vi "HART_read_modbus_register.vi"(0 "port number":refnum<visa-resource-name>, 1 "Max listen time\n(1000 ms)":u32=1000, 5 "address (array)":u8[](array[numeric]), 9 "MODBUS Reg.":u16=162, 11 "error IN":errorcluster, 12 "data type":T2(ring), 13 "Byte order":T1(ring)=enum."2-3-0-1") -> (2 "Data bytes":u8[](array[numeric]) format="%.0x", 3 "raw response":u8[](array[numeric]) format="%.0x", 4 "Unsigned 16 out":u16, 6 "unsigned 32 out":u32, 8 "raw write":u8[](array[numeric]) format="%.0x", 10 "floating point out":sgl format="%#.6f", 14 "coil value":u8, 15 "error out":errorcluster)   [LabVIEW 2016]
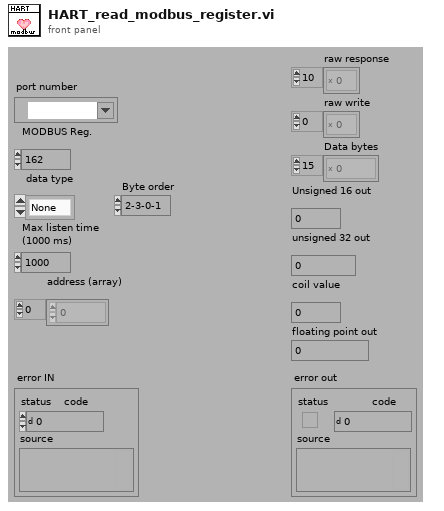
[diagram p1: front panel]
types:
  T1 = enum16{"0-1-2-3", "2-3-0-1", "1-0-3-2", "3-2-1-0"}
  T2 = enum16{"None", "Coil", "Uint16", "Uint32", "Float", "Undefined"}
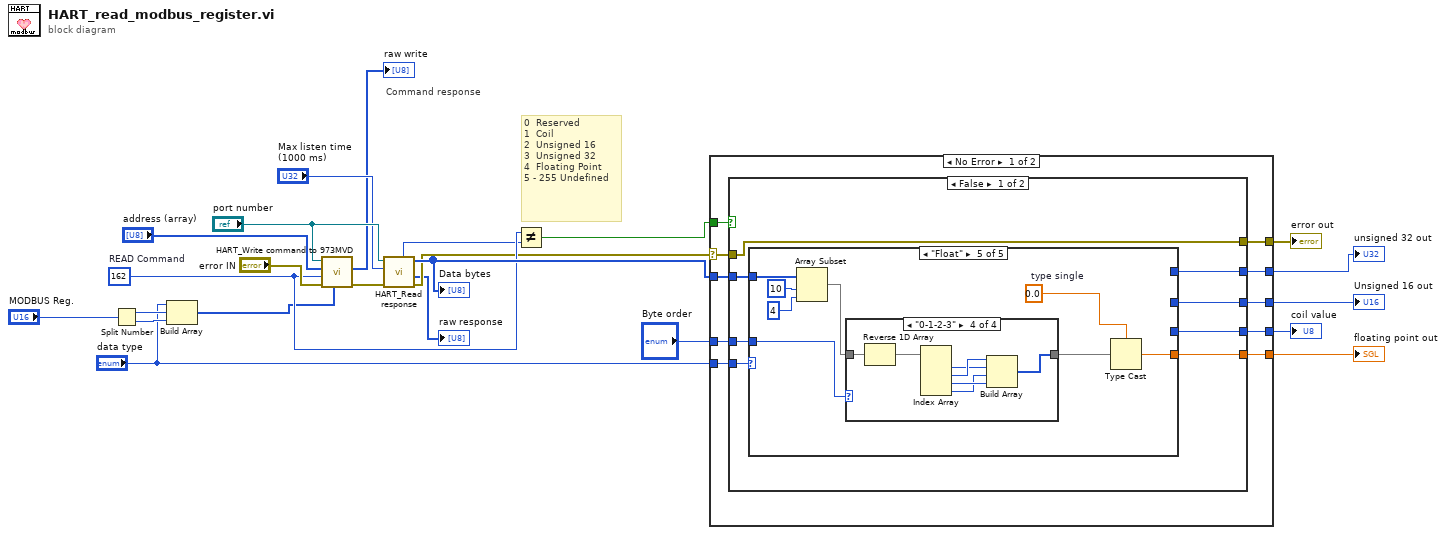
[diagram p0: block diagram]
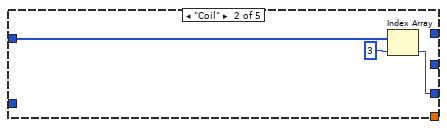
[diagram p3: hidden frame]
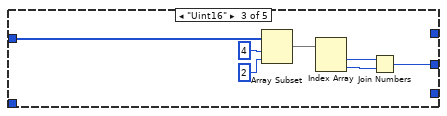
[diagram p4: hidden frame]
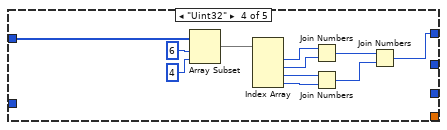
[diagram p5: hidden frame]
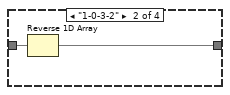
[diagram p7: hidden frame]
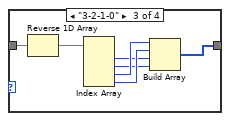
[diagram p8: hidden frame]
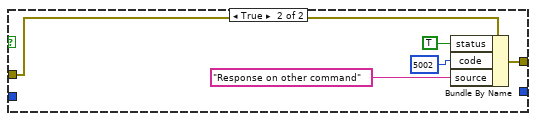
[diagram p9: hidden frame]
diagram:
  w19 = u8 162  # READ Command
  # "0\t\tReserved\n1\t\tCoil\n2\t\tUnsigned 16\n3\t\tUnsigned 32\n4\t\tFloating Point\n5 - 255\tUndefined"
  # "Command response"
  n1 = Split Number(x="MODBUS Reg.") -> (hi(x)=w13:u8, lo(x)=w12:u8)
  n2 = Build Array("data type", w13, w12) -> (w11:u16[])
  n3 = call "HART_Write command to 973MVD.vi"("data"=w11, "error in"="error IN", "READ Command"=w19, "address (array)"="address (array)", "resource name"="port number") -> ("error out"=w23:errorcluster, "appended array"=→"raw write":u8[])  [unwired: 5 in]
  n4 = call "HART_Read response.vi"("error in"=w23, "Max listen time\n(1000 ms)"="Max listen time\n(1000 ms)", "resource name"="port number") -> ("error out"=w16:errorcluster, "unsigned byte array"=→"raw response":u8[], "Data bytes"=w21:u8[], "Respons on\nCommand"=w18:u8)  [unwired: 3 in, 2 out]
  "Data bytes" <- w21
  n5 = Not Equal?(x=w19, y=w18) -> (x != y?=w20:bool)
  n6 = case shown="No Error" w16 {
    selector: w16 -> [w31 w93]
    tunnel: w21 -> [w33 _]
    tunnel: w20 -> [w32 _]
    tunnel: "data type" -> [w30 _]
    tunnel: [w29 w93] -> w10
    tunnel: [w28 _] -> w9
    tunnel: [w27 _] -> w8
    tunnel: [w26 _] -> w7
    tunnel: [w25 _] -> w6
    tunnel: "Byte order" -> [w24 _]
    frame No Error {
      n7 = case shown="False" w32 {
        tunnel: w33 -> [w40 _]
        tunnel: w31 -> [w39 w89]
        tunnel: [w39 w88] -> w29
        tunnel: w30 -> [w41 _]
        tunnel: [w38 _] -> w28
        tunnel: [w37 _] -> w27
        tunnel: [w36 _] -> w26
        tunnel: [w35 _] -> w25
        tunnel: w24 -> [w34 _]
        frame False {
          n8 = case shown="\"Float\"" w41 {
            tunnel: w40 -> [_ w44 w51 w62 w70]
            tunnel: [_ _ w45 _ _] -> w38
            tunnel: [_ _ _ w52 _] -> w37
            tunnel: [_ w42 _ _ _] -> w36
            tunnel: [_ _ _ _ w67] -> w35
            tunnel: w34 -> [_ _ _ _ w64]
            frame "None", Default {
            }
            frame "Coil" {
              n9 = Index Array(array=w44, index=3) -> (element=w42:u8)
            }
            frame "Uint16" {
              n10 = Array Subset(array=w51, index=4, length=2) -> (w48:u8[])
              n11 = Index Array(array=w48) -> (element #1=w47:u8, element #2=w46:u8)  [unwired: 2 in]
              n12 = Join Numbers(hi=w47, lo=w46) -> ((hi.lo)=w45:u16)
            }
            frame "Uint32" {
              n13 = Array Subset(array=w62, index=6, length=4) -> (w59:u8[])
              n14 = Index Array(array=w59) -> (element #1=w58:u8, element #2=w57:u8, element #3=w56:u8, element #4=w55:u8)  [unwired: 4 in]
              n15 = Join Numbers(hi=w58, lo=w57) -> ((hi.lo)=w54:u16)
              n16 = Join Numbers(hi=w56, lo=w55) -> ((hi.lo)=w53:u16)
              n17 = Join Numbers(hi=w54, lo=w53) -> ((hi.lo)=w52:u32)
            }
            frame "Float" {
              w66 = sgl 0.0  # type single
              n18 = Array Subset(array=w70, index=10, length=4) -> (w65:u8[])
              n19 = case shown="\"0-1-2-3\"" w64 {
                tunnel: w65 -> [w71 w73 w80 w87]
                tunnel: [w71 w72 w75 w86] -> w63
                frame "2-3-0-1" {
                }
                frame "1-0-3-2" {
                  n20 = Reverse 1D Array(array=w73) -> (reversed array=w72:u8[])
                }
                frame "3-2-1-0" {
                  n21 = Reverse 1D Array(array=w80) -> (reversed array=w74:u8[])
                  n22 = Index Array(array=w74) -> (element #1=w77:u8, element #2=w76:u8, element #3=w79:u8, element #4=w78:u8)  [unwired: 4 in]
                  n23 = Build Array(w79, w78, w77, w76) -> (w75:u8[])
                }
                frame "0-1-2-3" {
                  n24 = Reverse 1D Array(array=w87) -> (reversed array=w81:u8[])
                  n25 = Index Array(array=w81) -> (element #1=w84:u8, element #2=w85:u8, element #3=w83:u8, element #4=w82:u8)  [unwired: 4 in]
                  n26 = Build Array(w85, w84, w82, w83) -> (w86:u8[])
                }
              }
              n27 = Type Cast(type=w66, x=w63) -> (*(type *) &x=w67:sgl)
            }
          }
        }
        frame True {
          n28 = Bundle By Name(cluster=w89, "status"=TRUE ("Bundle Element"), "code"=5002 ("Bundle Element"), "source"="Response on other command" ("Bundle Element")) -> (w88:errorcluster)
        }
      }
    }
    frame Error {
    }
  }
  "error out" <- w10
  "Unsigned 16 out" <- w9
  "unsigned 32 out" <- w8
  "coil value" <- w7
  "floating point out" <- w6
